vi "visa学习和使用.vi"() -> ()   [LabVIEW 2022 SP3]
uses:
  <vilib>/Instr/_visa.llb/VISA Configure Serial Port (Instr).vi
panel:
  out "ENC":i32
  out "ADC":u16
  out "无符号字节数组":u8[](array[numeric])
  out "读取缓冲区 2":string
  in  "停止":bool
  in  "读取按钮":bool
  in  "写入按钮":bool
  in  "写入缓冲区":string
  out "读取缓冲区":string
  in  "VISA resource name":refnum<visa-resource-name> caption="VISA资源名称"
  in  "parity (0:none)":enum16{"None", "Odd", "Even", "Mark", "Space"}(ring) caption="奇偶（0:无）"
  in  "data bits (8)":u16=8 caption="数据比特(8)" min=5 max=8 step=1
  in  "baud rate (9600)":u32=9600 caption="波特率(9600)"
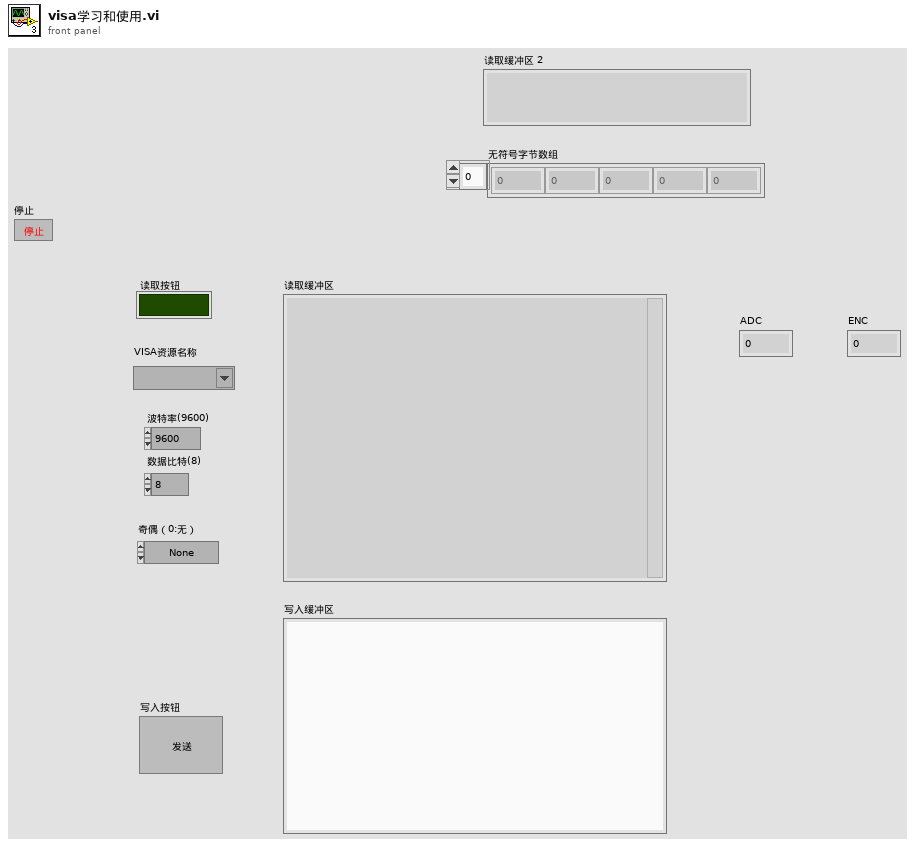
[diagram p1: front panel]
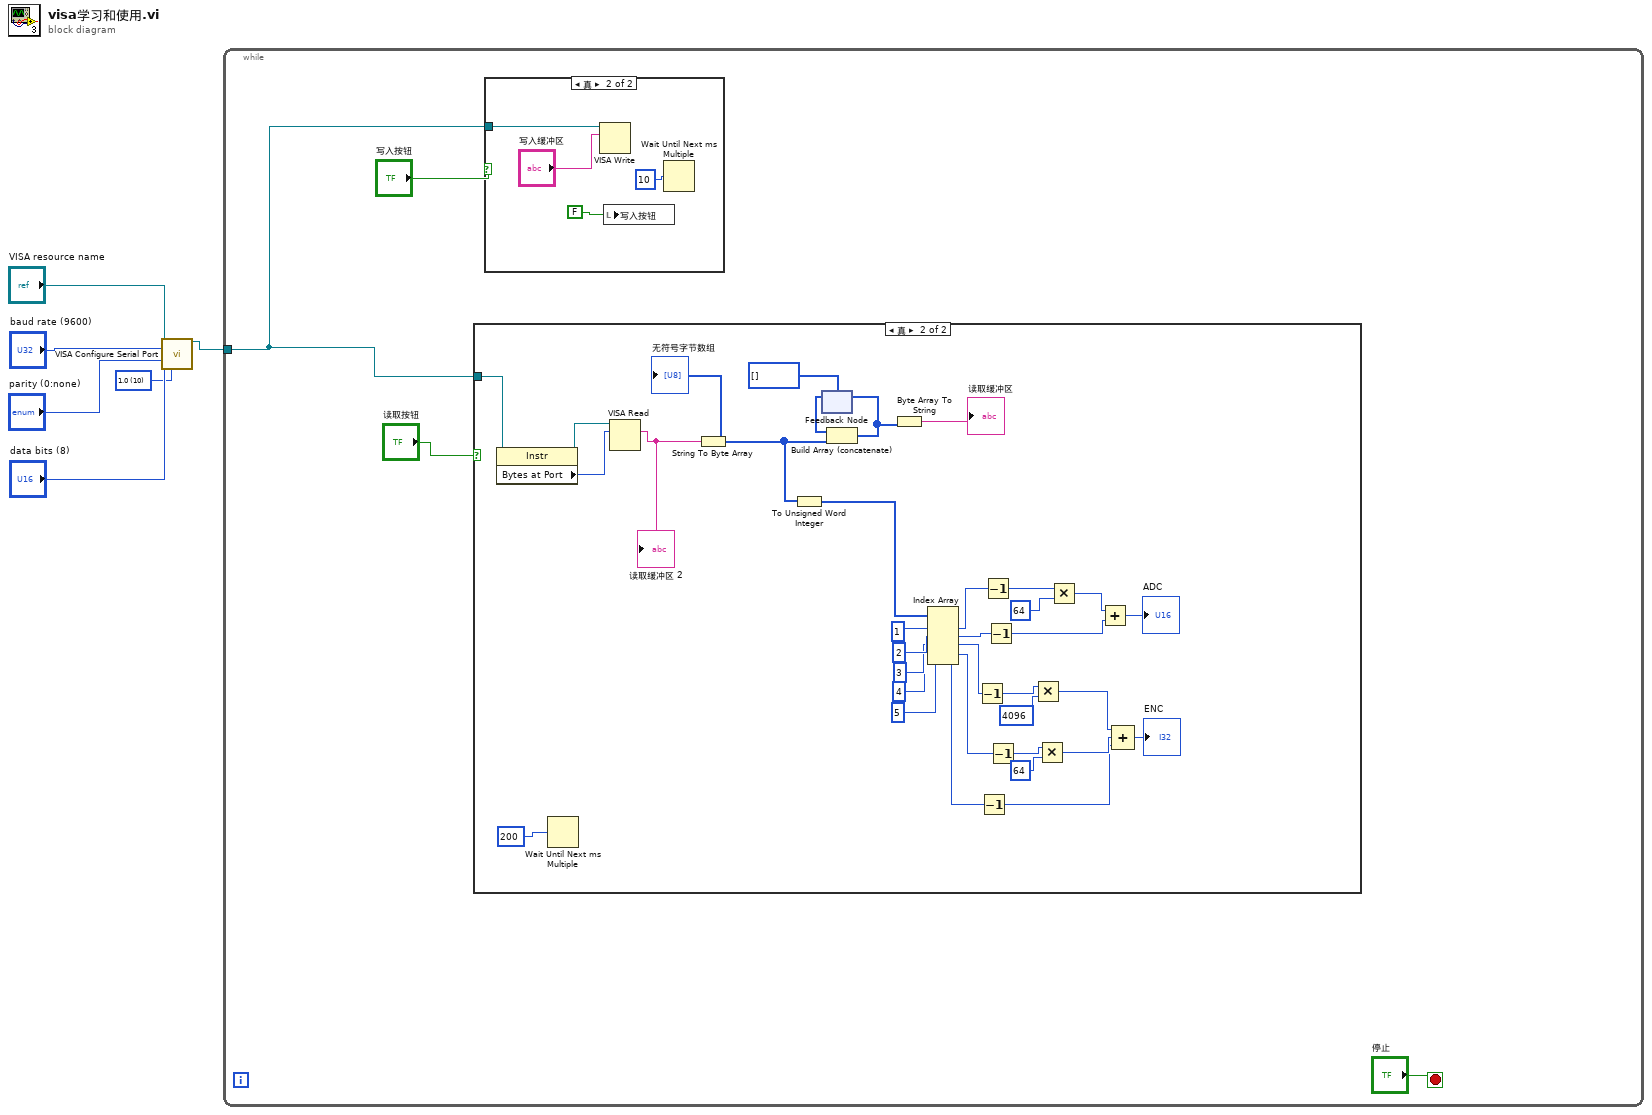
[diagram p0: block diagram]
diagram:
  w1 = u16 10 items=["1.0"=10, "1.5"=15, "2.0"=20] ("stop bits (10: 1 bit)")
  n1 = call-poly "VISA Configure Serial Port"("VISA resource name"="VISA resource name", "baud rate (9600)"="baud rate (9600)", "data bits (8)"="data bits (8)", "parity (0:none)"="parity (0:none)", "stop bits (10: 1 bit)"=w1) -> ("VISA resource name out"=w2:refnum<visa-resource-name>)  [unwired: 9 in, 1 out]
  n2 = while {
    tunnel: w2 -> [w7]
    stop <- "停止" stop-if-true
    n3 = case shown="真" "读取按钮" {
      tunnel: w7 -> [_ w13]
      frame False {
      }
      frame True {
        n4 = property class="Instr"(reference=w13) -> (reference out=w12:refnum<visa-resource-name>, "Bytes at Port"=w11:u32)  [unwired: 1 in, 1 out]
        n5 = Wait Until Next ms Multiple(millisecond multiple=u32 200 ("毫秒倍数")) -> ()  [unwired: 1 out]
        n6 = VISA Read(VISA resource name=w12, byte count=w11) -> (read buffer=w43:string)  [unwired: 1 in, 3 out]
        "读取缓冲区 2" <- w43
        n7 = String To Byte Array(string=w43) -> (unsigned byte array=w18:u8[])
        "无符号字节数组" <- w18
        n8 = To Unsigned Word Integer(number=w18) -> (unsigned 16bit integer=w16:u16[])
        n9 = feedback #1(u16[] []) -> (w42:u16[])
        n10 = Build Array (concatenate)(w42, w18) -> (w39:u16[])
        n11 = feedback-in #1(w39) -> ()
        n12 = Byte Array To String(unsigned byte array=w39) -> (string=→"读取缓冲区":string)
        n13 = Index Array(array=w16, index #1=1 ("索引"), index #2=2 ("索引"), index #3=3 ("索引"), index #4=4 ("索引"), index #5=5 ("索引")) -> (element #1=w23:u16, element #2=w22:u16, element #3=w21:u16, element #4=w20:u16, element #5=w19:u16)
        n14 = Decrement(x=w21) -> (x-1=w34:u16)
        n15 = Decrement(x=w19) -> (x-1=w28:u16)
        n16 = Decrement(x=w23) -> (x-1=w37:u16)
        n17 = Decrement(x=w22) -> (x-1=w35:u16)
        n18 = Decrement(x=w20) -> (x-1=w31:u16)
        n19 = Multiply(x=w34, y=4096) -> (x*y=w32:i32)
        n20 = Multiply(x=w31, y=u8 64) -> (x*y=w29:u16)
        n21 = Multiply(x=w37, y=u8 64) -> (x*y=w17:u16)
        n22 = Add(x=w17, y=w35) -> (x+y=→"ADC":u16)
        n23 = Compound Arithmetic op=ADD(w32, w29, w28) -> (→"ENC":i32)
      }
    }
    n24 = case shown="真" "写入按钮" {
      tunnel: w7 -> [_ w47]
      frame False {
      }
      frame True {
        n25 = VISA Write(VISA resource name=w47, write buffer="写入缓冲区") -> ()  [unwired: 1 in, 3 out]
        n26 = local write "写入按钮"(FALSE) -> ()
        n27 = Wait Until Next ms Multiple(millisecond multiple=u32 10 ("毫秒倍数")) -> ()  [unwired: 1 out]
      }
    }
  }
